vi "oef17.vi"() -> ()   [LabVIEW 2021]
uses:
  <vilib>/Utility/file.llb/Write Delimited Spreadsheet (I64).vi
  <vilib>/express/express arith-compare/Formula/XNode/ExpressFormulaBlockNode.xnode
panel:
  out "functions":i32[][](graph)
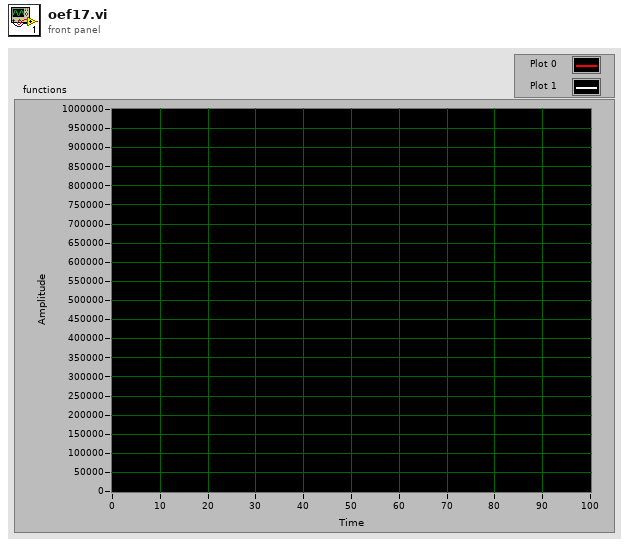
[diagram p1: front panel]
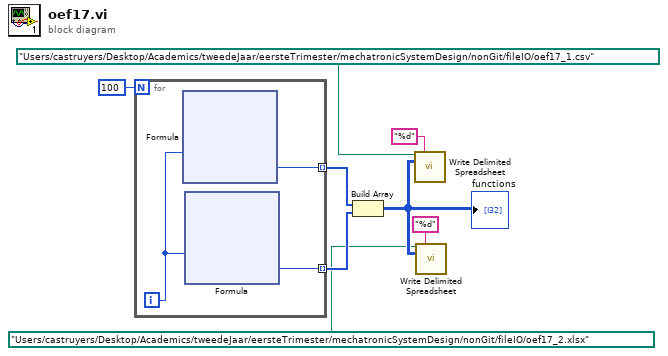
[diagram p0: block diagram]
diagram:
  n1 = for {
    N: 100 -> [_]
    tunnel: [w11] -> w6 mode=indexing
    tunnel: [w10] -> w5 mode=indexing
    i -> [w9]
    n2 = xnode "Formula"("x"=w9) -> ("Result"=w11:i32)  [unwired: 1 in, 1 out]
    n3 = xnode "Formula"("x"=w9) -> ("Result"=w10:i32)  [unwired: 1 in, 1 out]
  }
  n4 = Build Array(w6, w5) -> (w4:i32[][])
  "functions" <- w4
  n5 = call-poly <vilib>:"Write Delimited Spreadsheet.vi"("file path (dialog if empty)"=path "/Users/castruyers/Desktop/Academics/tweedeJaar/eersteTrimester/mechatronicSystemDesign/nonGit/fileIO/oef17_1.csv", "format (%d)"="%d", "2D data"=w4) -> ()  [unwired: 11 in, 2 out]
  n6 = call-poly <vilib>:"Write Delimited Spreadsheet.vi"("file path (dialog if empty)"=path "/Users/castruyers/Desktop/Academics/tweedeJaar/eersteTrimester/mechatronicSystemDesign/nonGit/fileIO/oef17_2.xlsx", "format (%d)"="%d", "2D data"=w4) -> ()  [unwired: 11 in, 2 out]
